vi "homework1.vi"() -> ()   [LabVIEW 2017]
panel:
  out "波形图表":dbl(graph)
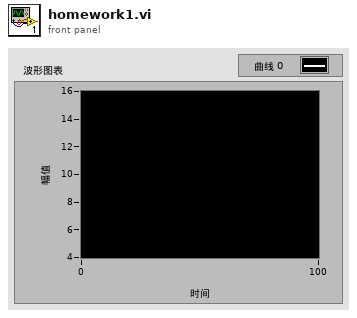
[diagram p1: front panel]
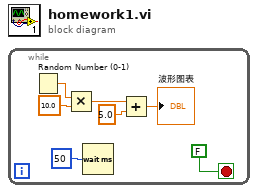
[diagram p0: block diagram]
diagram:
  n1 = while {
    stop <- FALSE stop-if-true
    n2 = Random Number (0-1)() -> (number: 0 to 1=w6:dbl)
    n3 = Multiply(x=w6, y=10.0) -> (x*y=w4:dbl)
    n4 = Wait (ms)(milliseconds to wait=u32 50 ("等待时间（毫秒）")) -> ()  [unwired: 1 out]
    n5 = Add(x=w4, y=5.0) -> (x+y=→"波形图表":dbl)
  }
